vi "Embed_Show.vi"(6 "Force?":bool=TRUE, 7 "Sub Panel":refnum<vi>, 8 "error in (no error)":errorcluster, 11 "EmbeddedSMO in":refnum<class "SMO.UI.Embedded.lvclass">) -> (0 "error out":errorcluster, 3 "EmbeddedSMO out":refnum<class "SMO.UI.Embedded.lvclass">)   [LabVIEW 2020, in "SMO.UI.Embedded.lvclass"]
uses:
  SMO.UI.Embedded.lvclass
  Typedefs/UI State.ctl
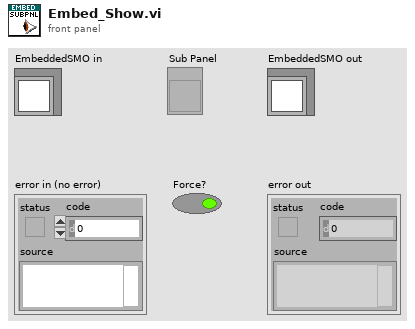
[diagram p1: front panel]
types:
  T1 = typedef "SMO.UI.Embedded.lvclass/UI State.ctl" = enum16{"unknown", "Opened", "Embedded", "Closed"}
  T2 = enum32{"Invalid", "Standard", "Closed", "Hidden", "Minimized", "Maximized"}
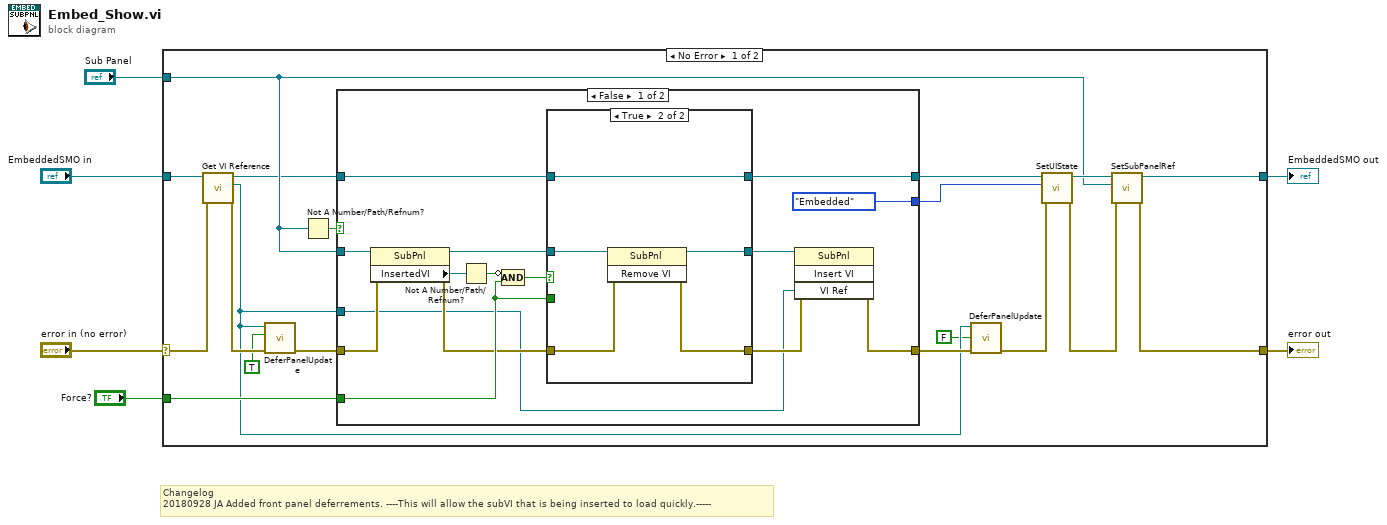
[diagram p0: block diagram]
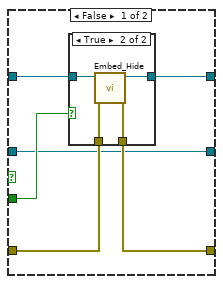
[diagram p2: hidden frame]
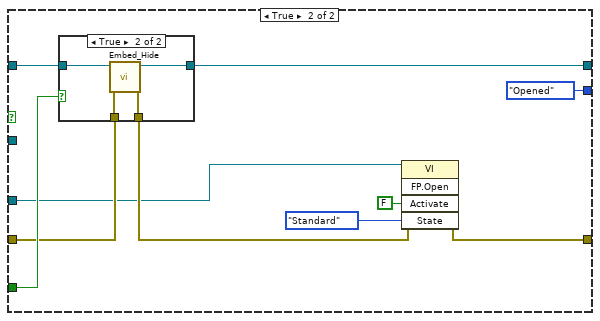
[diagram p4: hidden frame]
diagram:
  # "Changelog\n20180928 JA Added front panel deferrements. ----This will allow the subVI that is being inserted to load quickly.-----"
  n1 = case shown="No Error" "error in (no error)" {
    selector: "error in (no error)" -> [w15 w75]
    tunnel: [w17 w75] -> w5
    tunnel: [w20 w74] -> w1
    tunnel: "EmbeddedSMO in" -> [w16 w74]
    tunnel: "Force?" -> [w24 _]
    tunnel: "Sub Panel" -> [w18 _]
    frame No Error {
      n2 = call-dynamic "Get VI Reference.vi"("error in (no error)"=w15, "SMO UI"=w16) -> ("error out"=w13:errorcluster, "VI Reference"=w8:refnum<vi>, "SMO UI out"=w14:refnum<class "SMO.UI.Embedded.lvclass">)  [unwired: 7 in]
      n3 = call "DeferPanelUpdate.vi"("error in (no error)"=w13, "Defer Panel Updates"=TRUE ("Defer Updates?"), "VI in"=w8) -> ("error out"=w12:errorcluster)  [unwired: 8 in]
      n4 = Not A Number/Path/Refnum?(number/path/refnum=w18) -> (NaN/Path/Refnum?=w25:bool)
      n5 = case shown="False" w25 {
        tunnel: w14 -> [w34 w66]
        tunnel: [w33 w65] -> w23
        tunnel: w24 -> [w35 w67]
        tunnel: w8 -> [w26 w58]
        tunnel: w12 -> [w32 w64]
        tunnel: w18 -> [w40 _]
        tunnel: [w28 w60] -> w9
        tunnel: [UI_State."Embedded" ("UI State") UI_State."Opened" ("UI State")] -> w22
        frame False {
          n6 = property class="SubPnl"(reference=w40, error in=w32) -> (reference out=w36:refnum<vi>, error out=w31:errorcluster, "InsertedVI"=w37:refnum<vi>)
          n7 = Not A Number/Path/Refnum?(number/path/refnum=w37) -> (NaN/Path/Refnum?=w39:bool)
          n8 = Compound Arithmetic op=AND(invert w39, w35) -> (w38:bool)
          n9 = case shown="True" w38 {
            tunnel: w36 -> [w41 w57]
            tunnel: w35 -> [w46 _]
            tunnel: w34 -> [w45 w53]
            tunnel: [w44 w53] -> w33
            tunnel: w31 -> [w43 w54]
            tunnel: [w42 w55] -> w29
            tunnel: [w41 w56] -> w30
            frame False {
              n10 = case shown="True" w46 {
                tunnel: w45 -> [w47 w49]
                tunnel: [w47 w50] -> w44
                tunnel: w43 -> [w48 w52]
                tunnel: [w48 w51] -> w42
                frame False {
                }
                frame True {
                  n11 = call "Embed_Hide.vi"("error in (no error)"=w52, "EmbeddedSMO in"=w49) -> ("error out"=w51:errorcluster, "EmbeddedSMO out"=w50:refnum<class "SMO.UI.Embedded.lvclass">)  [unwired: 8 in]
                }
              }
            }
            frame True {
              n12 = invoke class="SubPnl" method="Remove VI"(reference=w57, error in=w54) -> (reference out=w56:refnum<vi>, error out=w55:errorcluster)  [unwired: 1 in, 1 out]
            }
          }
          n13 = invoke class="SubPnl" method="Insert VI"(reference=w30, error in=w29, "VI Ref"=w26) -> (error out=w28:errorcluster)  [unwired: 1 in, 3 out]
        }
        frame True {
          n14 = case shown="True" w67 {
            tunnel: w66 -> [w69 w70]
            tunnel: [w69 w71] -> w65
            tunnel: w64 -> [w68 w73]
            tunnel: [w68 w72] -> w63
            frame False {
            }
            frame True {
              n15 = call "Embed_Hide.vi"("error in (no error)"=w73, "EmbeddedSMO in"=w70) -> ("error out"=w72:errorcluster, "EmbeddedSMO out"=w71:refnum<class "SMO.UI.Embedded.lvclass">)  [unwired: 8 in]
            }
          }
          n16 = invoke class="VI" method="FP.Open"(reference=w58, error in=w63, "Activate"=FALSE ("Activate?"), "State"=T2."Standard" ("Front Panel Window:State")) -> (error out=w60:errorcluster)  [unwired: 1 in, 4 out]
        }
      }
      n17 = call "DeferPanelUpdate.vi"("error in (no error)"=w9, "Defer Panel Updates"=FALSE ("Defer Updates?"), "VI in"=w8) -> ("error out"=w10:errorcluster)  [unwired: 8 in]
      n18 = call "SetUIState.vi"("error in (no error)"=w10, "UI State"=w22, "EmbeddedSMO in"=w23) -> ("error out"=w19:errorcluster, "EmbeddedSMO out"=w21:refnum<class "SMO.UI.Embedded.lvclass">)  [unwired: 7 in]
      n19 = call "SetSubPanelRef.vi"("error in (no error)"=w19, "SubPanelReference"=w18, "EmbeddedSMO in"=w21) -> ("error out"=w17:errorcluster, "EmbeddedSMO out"=w20:refnum<class "SMO.UI.Embedded.lvclass">)  [unwired: 7 in]
    }
    frame Error {
    }
  }
  "error out" <- w5
  "EmbeddedSMO out" <- w1
